vi "Close.vi"(8 "error in (no error)":errorcluster, 11 "uService Template in":refnum<class "DAQ Sender.lvclass">) -> (0 "error out":errorcluster, 3 "uService Template out":refnum<class "DAQ Sender.lvclass">)   [LabVIEW 2020, in "CIRCUS_uServices.lvlib" / "DAQ Sender.lvlib" / "DAQ Sender.lvclass"]
uses:
  DAQ Sender.lvclass
  TALOS/TALOS_PPL.lvlibp/Father of all uServices/Father of all uServices/Father of all uServices.lvclass
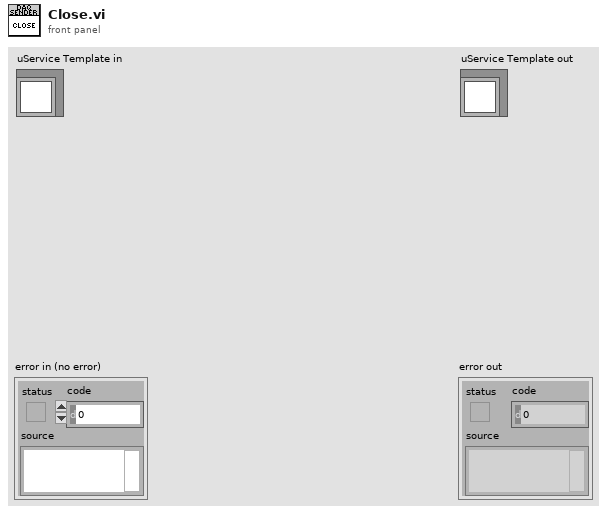
[diagram p1: front panel]
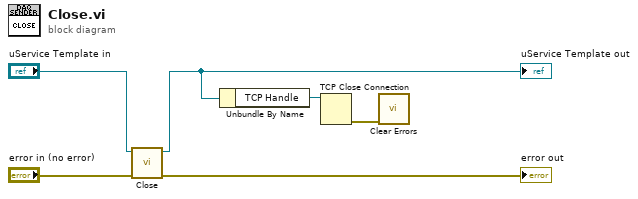
[diagram p0: block diagram]
diagram:
  n1 = call-parent "Close.vi"("error in (no error)"="error in (no error)", "uService Template in"="uService Template in") -> ("error out"=→"error out":errorcluster, "uService Template out"=w3:refnum<class "DAQ Sender.lvclass">)  [unwired: 8 in]
  "uService Template out" <- w3
  n2 = Unbundle By Name(w3) -> ("TCP Handle"=w2:refnum<k5>)
  n3 = TCP Close Connection(connection ID=w2) -> (error out=w1:errorcluster)  [unwired: 2 in, 1 out]
  n4 = call <vilib>:"Clear Errors.vi"("error in (no error)"=w1) -> ()  [unwired: 5 in, 2 out]
